vi "TTA_MATLAB_TX_TxAPCRTest_DetailedResults.vi"(8 "error in":errorcluster, 9 "ACPR Results":T1(array[cluster]), 10 "TestGroup":string, 11 "SubTest":string) -> (0 "error out":errorcluster, 3 "SubTestSuccess":dbl[](array[numeric]))   [LabVIEW 2016]
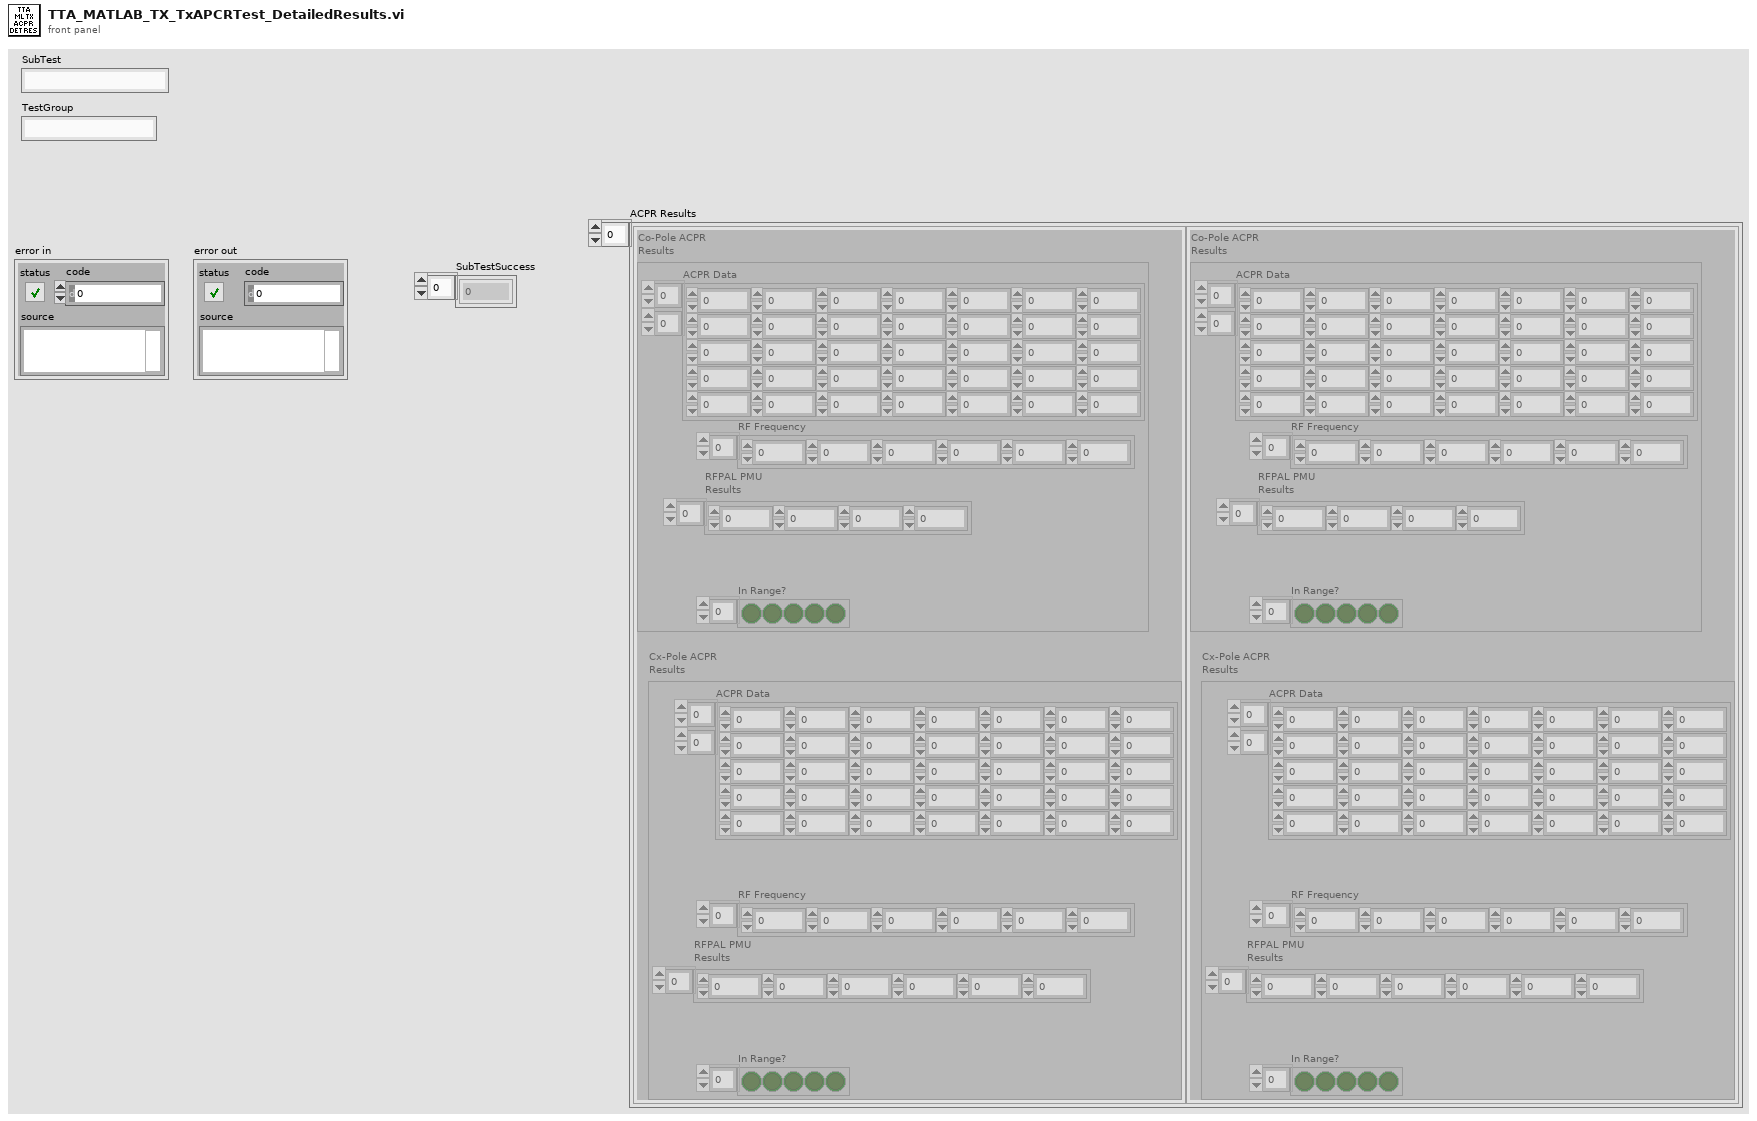
[diagram p1: front panel]
types:
  T1 = cluster{"Co-Pole ACPR\nResults":cluster{"ACPR Data":dbl[][], "RF Frequency":dbl[], "RFPAL PMU\nResults":dbl[], "In Range?":bool[]}, "Cx-Pole ACPR\nResults":cluster{"ACPR Data":dbl[][], "RF Frequency":dbl[], "RFPAL PMU\nResults":dbl[], "In Range?":bool[]}}[]
  T2 = cluster{"Co-Pole ACPR\nResults":cluster{"ACPR Data":dbl[][], "RF Frequency":dbl[], "RFPAL PMU\nResults":dbl[], "In Range?":bool[]}, "Cx-Pole ACPR\nResults":cluster{"ACPR Data":dbl[][], "RF Frequency":dbl[], "RFPAL PMU\nResults":dbl[], "In Range?":bool[]}}
  T3 = cluster{"ACPR Data":dbl[][], "RF Frequency":dbl[], "RFPAL PMU\nResults":dbl[], "In Range?":bool[]}
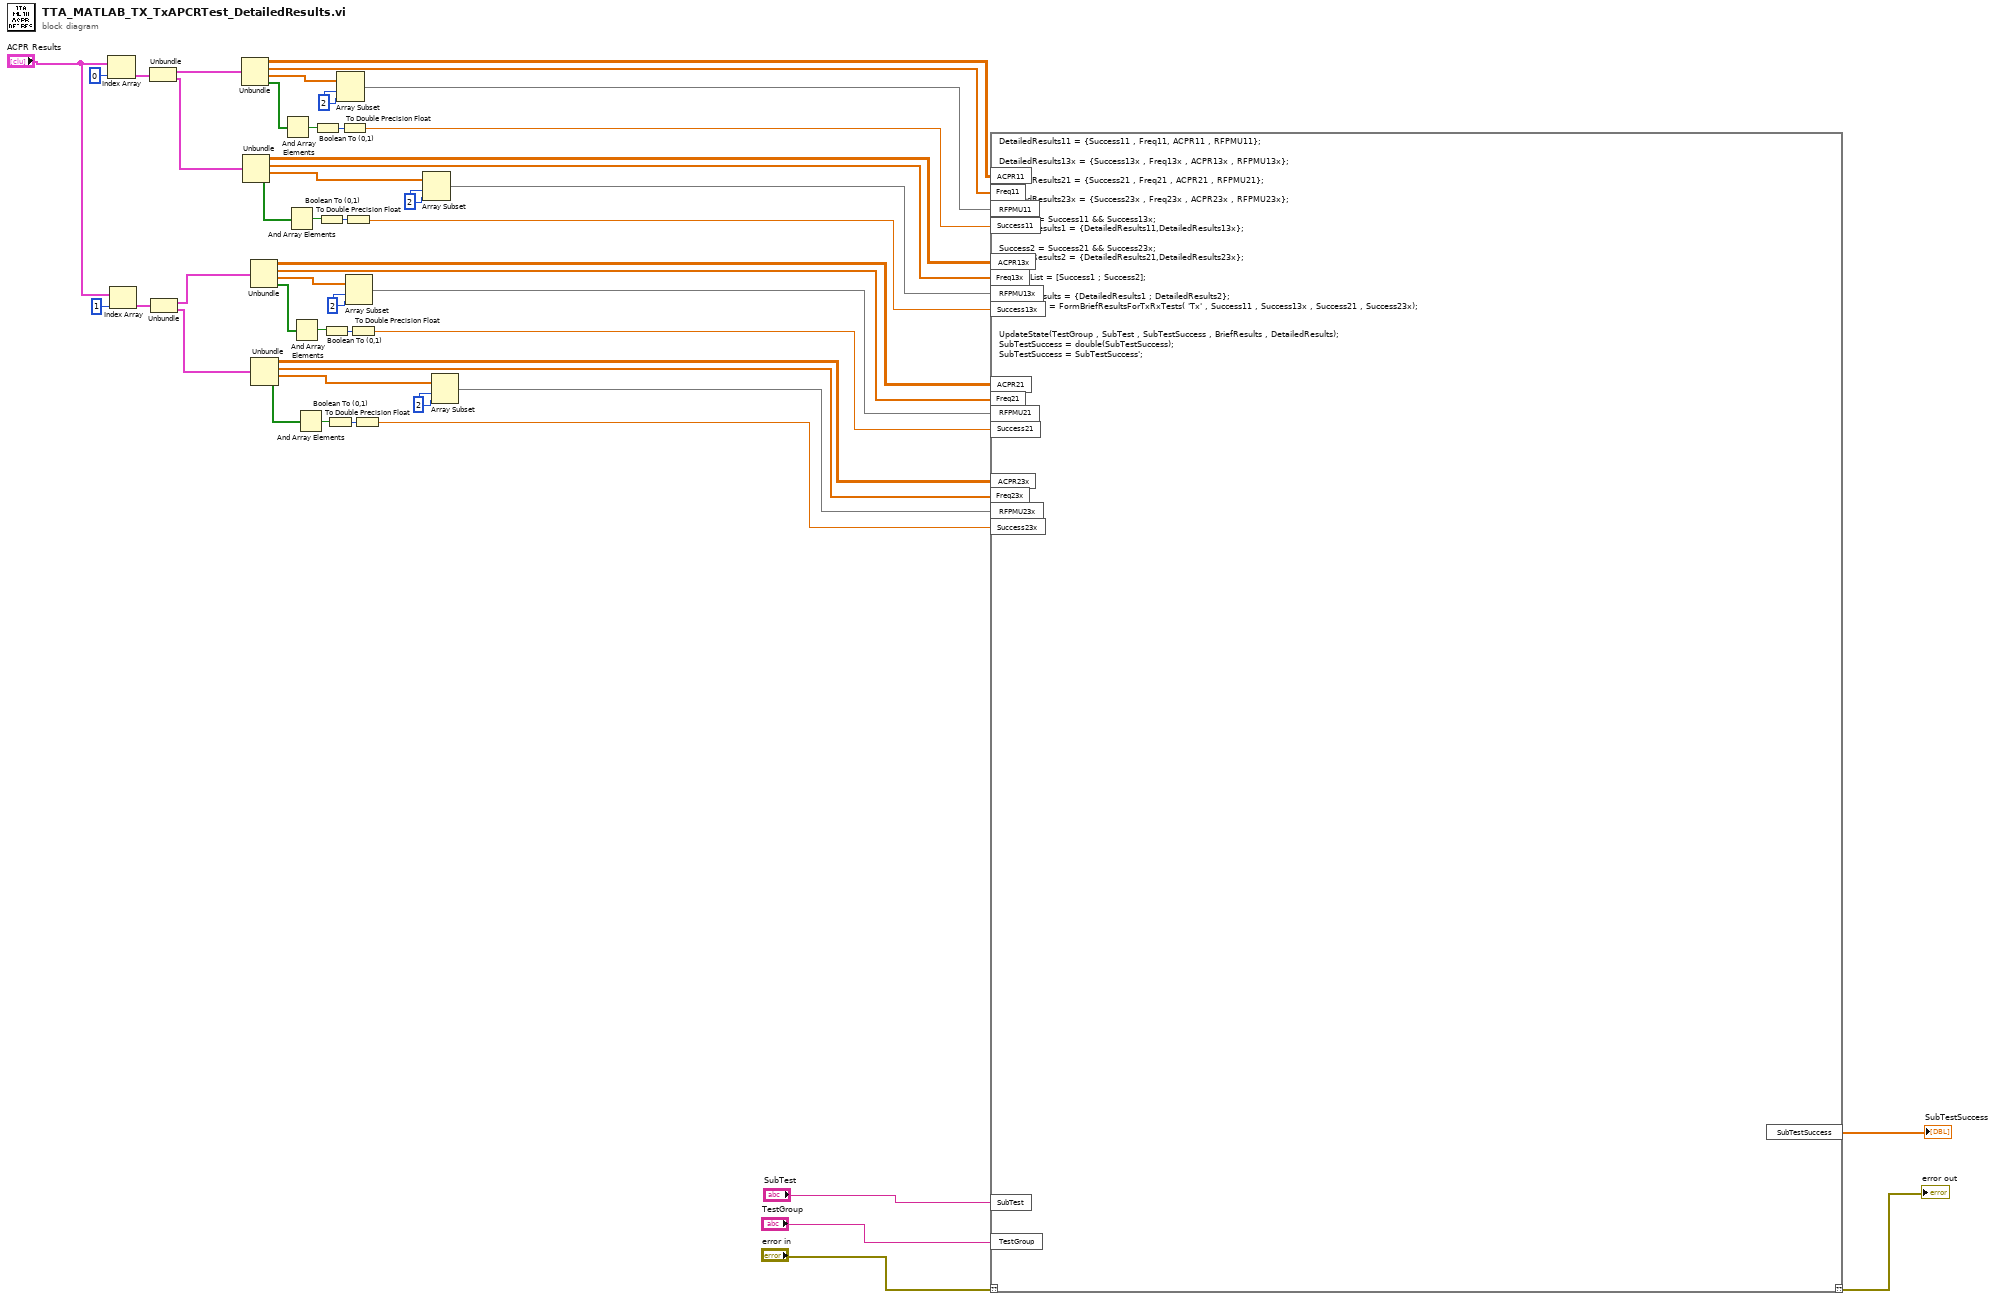
[diagram p0: block diagram]
diagram:
  w20 = 2 ("length")
  w17 = 2 ("length")
  w23 = 2 ("length")
  w29 = 2 ("length")
  (unwired) 1 ("index")
  (unwired) 0 ("index")
  (unwired) 1 ("index")
  (unwired) 0 ("index")
  (unwired) 1 ("index")
  (unwired) 0 ("index")
  (unwired) 1 ("index")
  (unwired) 0 ("index")
  n1 = Index Array(array="ACPR Results", index=0) -> (element=w37:T2)
  n2 = Index Array(array="ACPR Results", index=1) -> (element=w36:T2)
  n3 = Unbundle(w37) -> ("Co-Pole ACPR\nResults"=w35:T3, "Cx-Pole ACPR\nResults"=w33:T3)
  n4 = Unbundle(w36) -> ("Co-Pole ACPR\nResults"=w10:T3, "Cx-Pole ACPR\nResults"=w9:T3)
  n5 = Unbundle(w35) -> ("ACPR Data"=w31:dbl[][], "RF Frequency"=w30:dbl[], "RFPAL PMU\nResults"=w28:dbl[], "In Range?"=w34:bool[])
  n6 = Unbundle(w33) -> ("ACPR Data"=w26:dbl[][], "RF Frequency"=w25:dbl[], "RFPAL PMU\nResults"=w24:dbl[], "In Range?"=w32:bool[])
  n7 = Unbundle(w10) -> ("ACPR Data"=w8:dbl[][], "RF Frequency"=w7:dbl[], "RFPAL PMU\nResults"=w18:dbl[], "In Range?"=w15:bool[])
  n8 = Unbundle(w9) -> ("ACPR Data"=w4:dbl[][], "RF Frequency"=w3:dbl[], "RFPAL PMU\nResults"=w19:dbl[], "In Range?"=w16:bool[])
  n9 = And Array Elements(Boolean array=w34) -> (logical AND=w44:bool)
  n10 = And Array Elements(Boolean array=w32) -> (logical AND=w40:bool)
  n11 = And Array Elements(Boolean array=w15) -> (logical AND=w11:bool)
  n12 = And Array Elements(Boolean array=w16) -> (logical AND=w14:bool)
  n13 = Boolean To (0,1)(Boolean=w44) -> (0, 1=w43:i16)
  n14 = Boolean To (0,1)(Boolean=w40) -> (0, 1=w41:i16)
  n15 = Boolean To (0,1)(Boolean=w11) -> (0, 1=w12:i16)
  n16 = Boolean To (0,1)(Boolean=w14) -> (0, 1=w13:i16)
  n17 = Array Subset(array=w28, index=w29, length=w29) -> (w27:dbl[])
  n18 = To Double Precision Float(number=w43) -> (double precision float=w42:dbl)
  n19 = To Double Precision Float(number=w41) -> (double precision float=w21:dbl)
  n20 = Array Subset(array=w18, index=w17, length=w17) -> (w6:dbl[])
  n21 = To Double Precision Float(number=w12) -> (double precision float=w5:dbl)
  n22 = To Double Precision Float(number=w13) -> (double precision float=w1:dbl)
  n23 = Array Subset(array=w24, index=w23, length=w23) -> (w22:dbl[])
  n24 = Array Subset(array=w19, index=w20, length=w20) -> (w2:dbl[])
  n25 = script code="DetailedResults11 = {Success11 , Freq11, ACPR11 , RFPMU11};\n\nDetailedResults13x = {Success13x , Freq13x , ACPR13x , RFPMU13x};\n\nDetailedResults21 = {Success21 , Freq21 , ACPR21 , RFPMU21};\n\nDetailedResults23x = {Success23x , Freq23x , ACPR23x , RFPMU23x};\n\nSuccess1 = Success11 && Success13x;\nDetailedResults1 = {DetailedResults11,DetailedResults13x};\n\nSuccess2 = Success21 && Success23x;\nDetailedResults2 = {DetailedResults21,DetailedResults23x};\n\nSuccessList = [Success1 ; Success2];\n\nDetailedResults = {DetailedResults1 ; DetailedResults2};\nBriefResults = FormBriefResultsForTxRxTests( 'Tx' , Success11 , Success13x , Success21 , Success23x);\n                                          \n\nUpdateState(TestGroup , SubTest , SubTestSuccess , BriefResults , DetailedResults);\nSubTestSuccess = double(SubTestSuccess);\nSubTestSuccess = SubTestSuccess';"("??"="error in", "SubTest"="SubTest", "TestGroup"="TestGroup", "Success11"=w42, "ACPR11"=w31, "Freq11"=w30, "RFPMU11"=w27, "ACPR13x"=w26, "Freq13x"=w25, "RFPMU13x"=w22, "Success13x"=w21, "Success21"=w5, "ACPR21"=w8, "Freq21"=w7, "RFPMU21"=w6, "Success23x"=w1, "ACPR23x"=w4, "Freq23x"=w3, "RFPMU23x"=w2) -> ("??"=→"error out":errorcluster, "SubTestSuccess"=→"SubTestSuccess":dbl[])
